vi "DT_Find Next Triangulation.vi"(8 "cur point":i32, 9 "next triangle in":i32, 10 "Triangles In":i32[][](array[numeric]), 11 "Points In":cluster{"x":dbl, "y":dbl, "index":i32}[](array[cluster])) -> (0 "next point":i32, 1 "next triangle out":i32, 2 "Triangles Out":i32[][](array[numeric]), 3 "Points Out":cluster{"x":dbl, "y":dbl, "index":i32}[](array[cluster]), 4 "error":i32)   [LabVIEW 2017, in "NI_AAL_Geometry.lvlib"]
uses:
  <vilib>/Analysis/NI_AAL_Geometry.lvlib
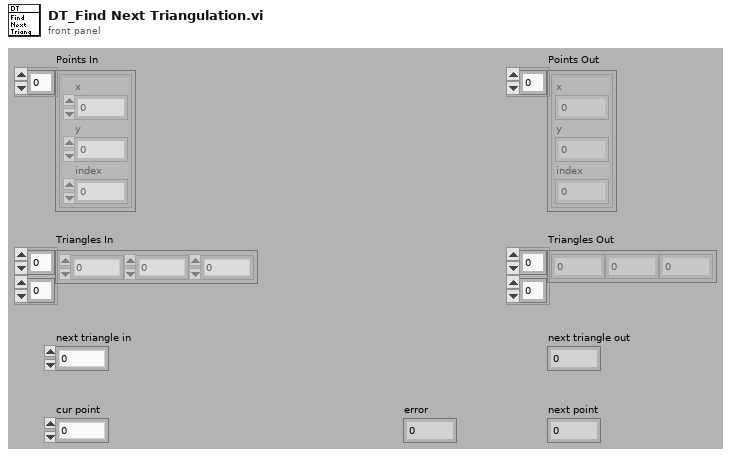
[diagram p1: front panel]
types:
  T1 = typedef "NI_AAL_Geometry.lvlib/DT_Find Next Triangulation_Data.ctl" = cluster{"cur point":i32, "cur triangle":i32, "cur local idx":i32, "base point":i32, "base triangle":i32, "base local idx":i32, "Candidate Triangles":i32[], "Candidate Point Idx":i32[]}
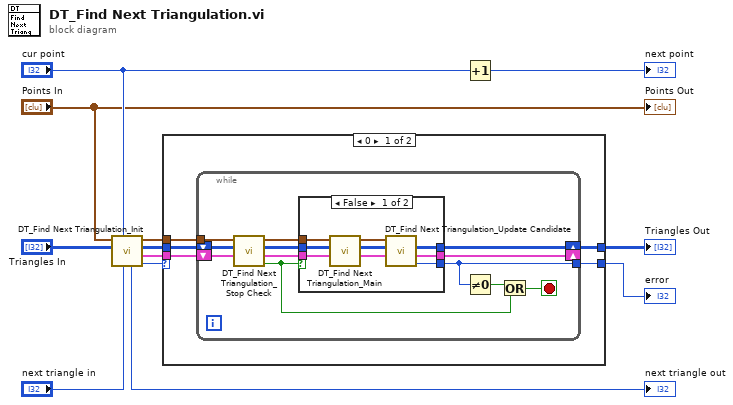
[diagram p0: block diagram]
diagram:
  n1 = call <vilib>:"DT_Find Next Triangulation_Init.vi"("next triangle in"="next triangle in", "cur point"="cur point", "Triangles In"="Triangles In", "Points In"="Points In") -> ("error"=w2:i32, "Data"=w10:T1, "Triangles Out"=w8:i32[][], "Points Out"=w9:cluster{"x":dbl, "y":dbl, "index":i32}[], "next triangle out"=→"next triangle out":i32)  [unwired: 2 in, 1 out]
  n2 = case shown="0" w2 {
    selector: w2 -> [_ w41]
    tunnel: [w17 _] -> w11
    tunnel: w10 -> [w16 _]
    tunnel: w9 -> [w15 _]
    tunnel: w8 -> [w14 _]
    tunnel: [w13 w41] -> w1
    frame 0 {
      n3 = while {
        shift-right: [w26] -> w17
        shift-left: w14 -> [w23]
        shift-right: [w25] -> _
        shift-left: w16 -> [w22]
        tunnel: w15 -> [w24]
        tunnel: [w21] -> w13
        stop <- w18 stop-if-true
        n4 = call <vilib>:"DT_Find Next Triangulation_Stop Check.vi"("Data In"=w22, "Triangles In"=w23, "Points In"=w24) -> ("stop?"=w19:bool, "Data Out"=w27:T1, "Triangles Out"=w28:i32[][], "Points Out"=w29:cluster{"x":dbl, "y":dbl, "index":i32}[])  [unwired: 5 out]
        n5 = case shown="False" w19 {
          tunnel: w29 -> [w36 _]
          tunnel: w28 -> [w33 w40]
          tunnel: w27 -> [w32 w39]
          tunnel: [w38 w40] -> w26
          tunnel: [w37 w39] -> w25
          tunnel: [w30 _] -> w21
          frame False {
            n6 = call <vilib>:"DT_Find Next Triangulation_Main.vi"("Data In"=w32, "Triangles In"=w33, "Points In"=w36) -> ("Data Out"=w31:T1, "Triangles Out"=w34:i32[][], "Points Out"=w35:cluster{"x":dbl, "y":dbl, "index":i32}[])  [unwired: 3 in, 3 out]
            n7 = call <vilib>:"DT_Find Next Triangulation_Update Candidate.vi"("Data In"=w31, "Triangles In"=w34, "Points In"=w35) -> ("error"=w30:i32, "Data Out"=w37:T1, "Triangles Out"=w38:i32[][])  [unwired: 6 out]
          }
          frame True {
          }
        }
        n8 = Not Equal To 0?(x=w21) -> (x != 0?=w20:bool)
        n9 = Or(x=w20, y=w19) -> (x .or. y?=w18:bool)
      }
    }
    frame 1, Default {
    }
  }
  "Triangles Out" <- w11
  "error" <- w1
  n10 = Increment(x="cur point") -> (x+1=→"next point":i32)
  "Points Out" <- "Points In"
